vi "UnitTest-UpdateData.vi"(8 "error in":errorcluster, 10 "LV Data":T1={"Numeric Data"=1, "Float Data"=1.0, "String Data"="This is string", "Enum Data"=enum."Enum Item 2", "Array Data"=[1234, 2345, 3456, 4567]}, 11 "TableLogger Config":T2={"TableLogger"=enum."CSV Logger", "DB File Path"=path "C:/LogAnyLVdata/Test.csv", "DB Backup Config"={"Directory"=path "C:/LogAnyLVdata/dBbackup", "UTC Time Format"=FALSE, "On Launch"=TRUE, "Interval (Hours)"=24.0, "Size Multiples (Bytes)"=500}}) -> (0 "error out":errorcluster)   [LabVIEW 2014]
uses:
  <vilib>/addons/_JKI Toolkits/Caraya/classes/Test/Test.lvclass
  TableLogger_Actor/TableLogger_Actor/TableLogger_Actor.lvclass
  <vilib>/addons/_JKI Toolkits/Caraya/classes/Assert/Assert.lvclass
  <vilib>/ActorFramework/Stop Msg/Stop Msg.lvclass
  <vilib>/Utility/file.llb/Read Delimited Spreadsheet (string).vi
  TableLogger_Actor/TableLoggerTypes.ctl
  TableLogger_Actor/TableLogger_Actor.lvlib
  TableLogger_Actor/TableLoggerConfig.ctl
  TableLogger_Actor/TableLoggerDataCluster.ctl
  TableLogger_Actor/TableLoggerBackupConfig.ctl
panel:
  # "Connector Pane"
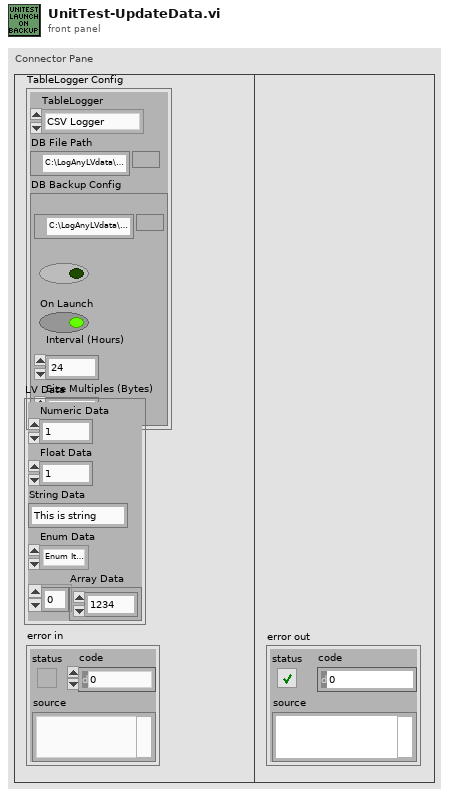
[diagram p1: front panel]
types:
  T1 = typedef "TableLogger_Actor.lvlib/TableLoggerDataCluster.ctl" = cluster{"Numeric Data":i32, "Float Data":dbl, "String Data":string, "Enum Data":enum16{"Enum Item 1", "Enum Item 2"}, "Array Data":i32[]}
  T2 = typedef "TableLogger_Actor.lvlib/TableLoggerConfig.ctl" = cluster{"TableLogger":T3, "DB File Path":path, "DB Backup Config":T4}
  T3 = typedef "TableLogger_Actor.lvlib/TableLoggerTypes.ctl" = enum16{"CSV Logger", "SQLite Logger"}
  T4 = typedef "TableLogger_Actor.lvlib/TableLoggerBackupConfig.ctl" = cluster{"Directory":path, "UTC Time Format":bool, "On Launch":bool, "Interval (Hours)":dbl, "Size Multiples (Bytes)":i32}
  T5 = typedef "File Info Record__ogtk.ctl" = cluster{"type":string, "creator":string, "permissions":i32, "data size":i32, "res size":i32, "creation date":u32, "modification date":u32, "bFolder":bool, "bInvisible":bool, "location":cluster{"vertical":i16, "horizontal":i16}, "owner":string, "group":string}
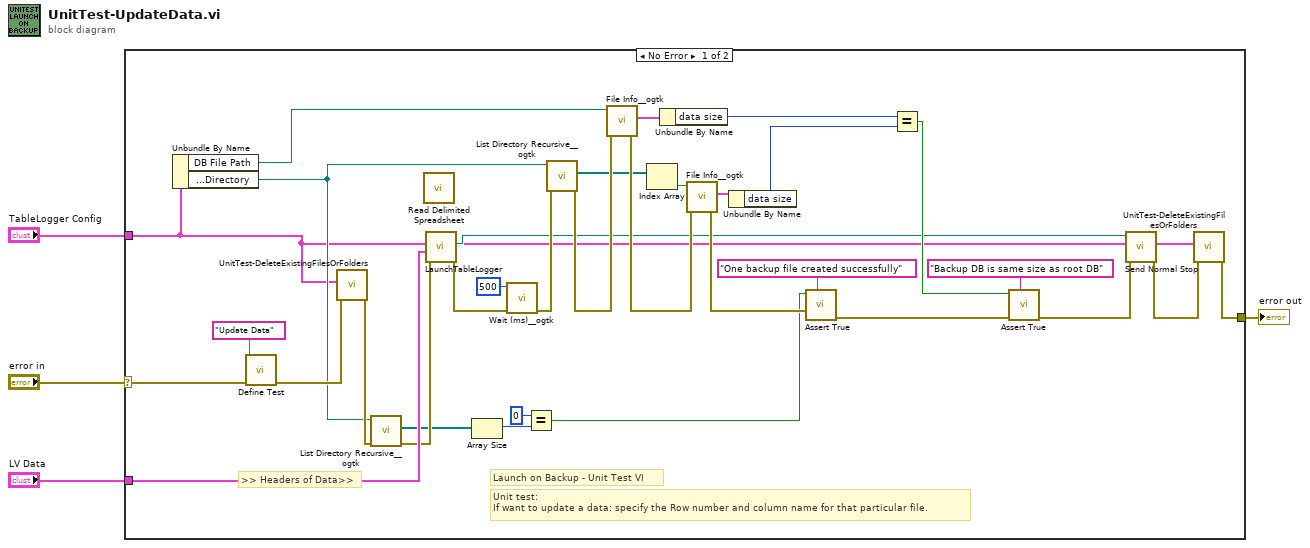
[diagram p0: block diagram]
diagram:
  n1 = case shown="No Error" "error in" {
    selector: "error in" -> [w36 w38]
    tunnel: "LV Data" -> [w37 _]
    tunnel: "TableLogger Config" -> [w5 _]
    tunnel: [w8 w38] -> w2
    frame No Error {
      # "Unit test:\nIf want to update a data: specify the Row number and column name for that particular file."
      # "Launch on Backup - Unit Test VI"
      # ">> Headers of Data>>"
      n2 = Unbundle By Name(w5) -> ("DB File Path"=w7:path, "DB Backup Config.Directory"=w6:path)
      n3 = call <vilib>:"Define Test.vi"("error in (no error)"=w36, "Label (VI Title)"="Update Data") -> ("error out"=w12:errorcluster)  [unwired: 9 in]
      n4 = call "UnitTest-DeleteExistingFilesOrFolders.vi"("error in (no error)"=w12, "Config IN"=w5) -> ("error out"=w32:errorcluster)  [unwired: 9 in]
      n5 = call <userlib>:"List Directory Recursive__ogtk.vi"("error in (no error)"=w32, "Path"=w6) -> ("error out"=w30:errorcluster, "file paths"=w29:path[])  [unwired: 6 in, 2 out]
      n6 = call-poly <vilib>:"Read Delimited Spreadsheet.vi"() -> ()  [unwired: 10 in, 6 out]
      n7 = call "LaunchTableLogger.vi"("error in (no error)"=w30, "Data Cluster (for Headers)"=w37, "TableLogger Config"=w5) -> ("error out"=w27:errorcluster, "TableLogger Actor's Enqueuer"=w10:refnum<class "Message Enqueuer.lvclass">)  [unwired: 5 in, 2 out]
      n8 = Array Size(array=w29) -> (size(s)=w14:i32)
      n9 = call <userlib>:"Wait (ms)__ogtk.vi"("error in (no error)"=w27, "milliseconds to wait"=u32 500) -> ("error out"=w28:errorcluster)  [unwired: 8 in, 1 out]
      n10 = Equal?(x=0, y=w14) -> (x = y?=w22:bool)
      n11 = call <userlib>:"List Directory Recursive__ogtk.vi"("error in (no error)"=w28, "Path"=w6) -> ("error out"=w33:errorcluster, "file paths"=w18:path[])  [unwired: 6 in, 2 out]
      n12 = call <userlib>:"File Info__ogtk.vi"("error in (no error)"=w33, "file"=w7) -> ("error out"=w34:errorcluster, "file info"=w21:T5)  [unwired: 4 in, 1 out]
      n13 = Index Array(array=w18) -> (element=w19:path)  [unwired: 1 in]
      n14 = Unbundle By Name(w21) -> ("data size"=w23:i32)
      n15 = call <userlib>:"File Info__ogtk.vi"("error in (no error)"=w34, "file"=w19) -> ("error out"=w35:errorcluster, "file info"=w20:T5)  [unwired: 4 in, 1 out]
      n16 = Unbundle By Name(w20) -> ("data size"=w24:i32)
      n17 = call <vilib>:"Assert True.vi"("Label"="One backup file created successfully", "error in (no error)"=w35, "True?"=w22) -> ("error out"=w16:errorcluster)  [unwired: 8 in]
      n18 = Equal?(x=w23, y=w24) -> (x = y?=w25:bool)
      n19 = call <vilib>:"Assert True.vi"("Label"="Backup DB is same size as root DB", "error in (no error)"=w16, "True?"=w25) -> ("error out"=w13:errorcluster)  [unwired: 8 in]
      n20 = call <vilib>:"Send Normal Stop.vi"("error in (no error)"=w13, "Message Enqueuer"=w10) -> ("error out"=w9:errorcluster)  [unwired: 9 in]
      n21 = call "UnitTest-DeleteExistingFilesOrFolders.vi"("error in (no error)"=w9, "Config IN"=w5) -> ("error out"=w8:errorcluster)  [unwired: 9 in]
    }
    frame Error {
    }
  }
  "error out" <- w2
